vi "Add 0 to non-empty array.vi"(1 "Voltages in":dbl[](array[numeric])) -> (0 "Voltages out":dbl[](array[numeric]))   [LabVIEW 2013]
doc: "If given array is not empty, adds an element of 0 to it."
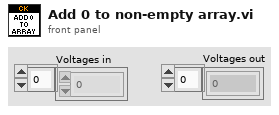
[diagram p1: front panel]
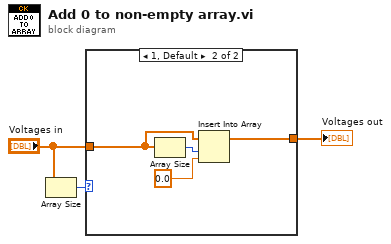
[diagram p0: block diagram]
diagram:
  n1 = Array Size(array="Voltages in") -> (size(s)=w2:i32)
  n2 = case shown="1, Default" w2 {
    tunnel: [w4 w8] -> w3
    tunnel: "Voltages in" -> [w4 w7]
    frame 0 {
    }
    frame 1, Default {
      n3 = Array Size(array=w7) -> (size(s)=w5:i32)
      n4 = Insert Into Array(array=w7, index=w5, new element=0.0 ("new element/subarray")) -> (w8:dbl[])
    }
  }
  "Voltages out" <- w3
